vi "CAMcalibrator.vi"() -> ()   [LabVIEW 2011]
uses:
  <vilib>/userDefined/High Color/IMAQdx.ctl
  <vilib>/vision/driver/NI_Vision_Acquisition_Software.lvlib
panel:
  out "I (mA)":dbl
  out "Image":T1(plugin-control)
  in  "APTLaser":refnum<k7>(container) caption="Resume"
  in  "LaserON":bool
  in  "Set Current at:":sgl=70.0 caption="mA"
  in  "Parada Total":bool
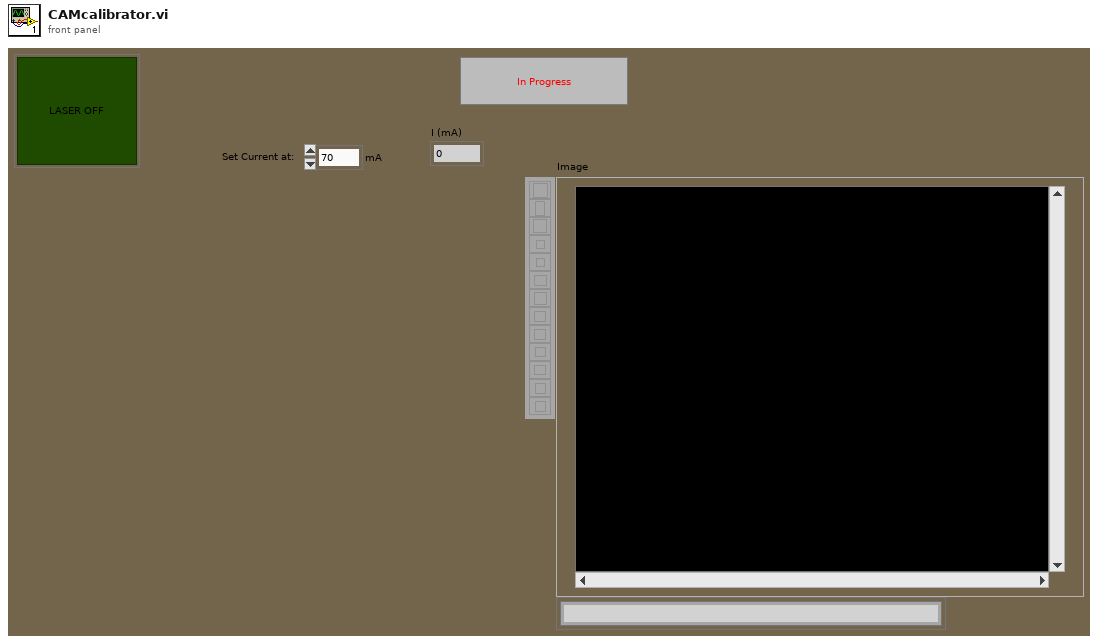
[diagram p1: front panel]
types:
  T1 = typedef "IMAQ Image.ctl" = refnum<image>
  T2 = typedef "IMAQdx.ctl" = refnum<k21>
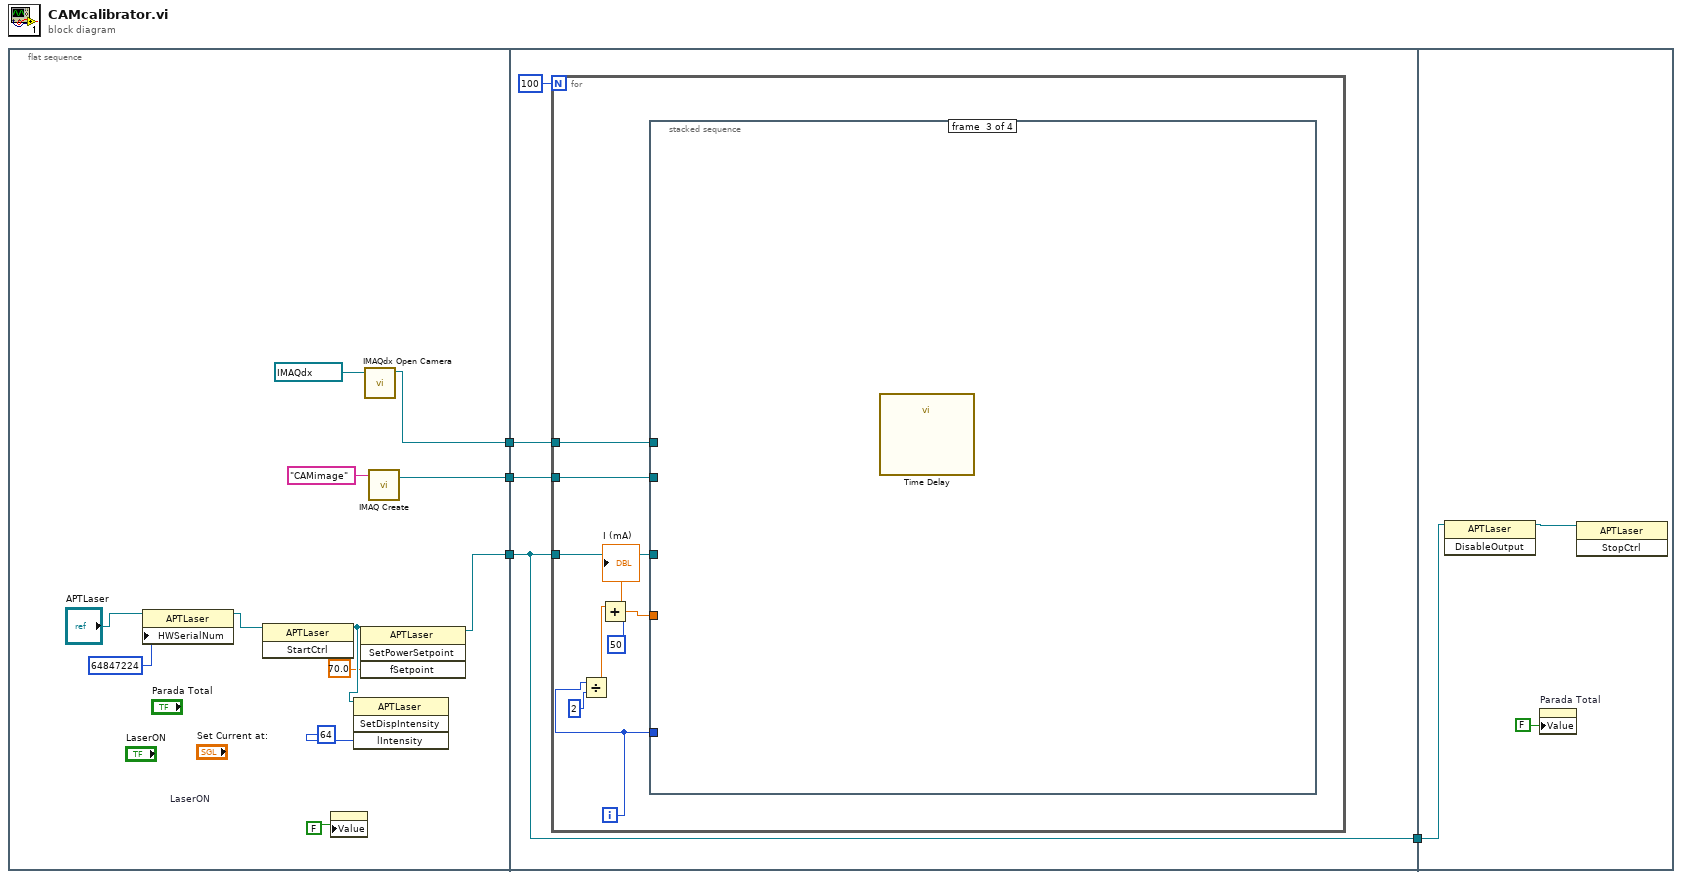
[diagram p0: block diagram]
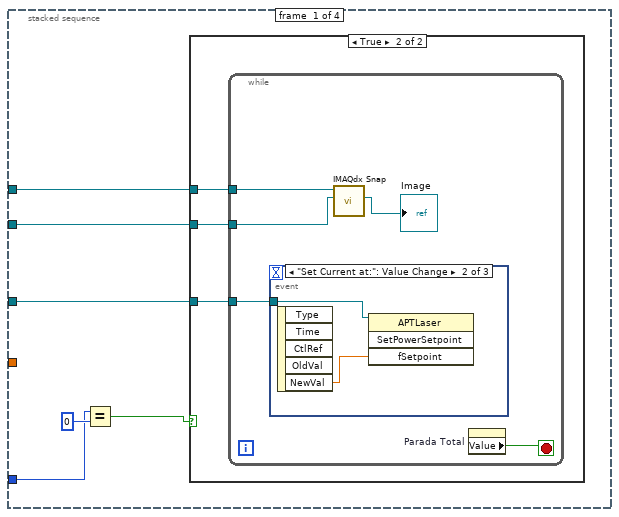
[diagram p2: hidden frame]
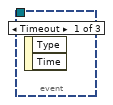
[diagram p4: hidden frame]
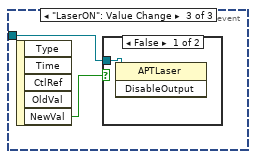
[diagram p5: hidden frame]
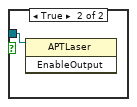
[diagram p6: hidden frame]
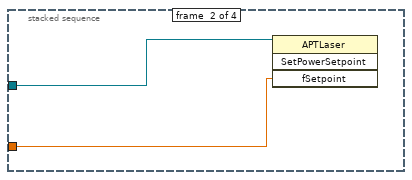
[diagram p7: hidden frame]
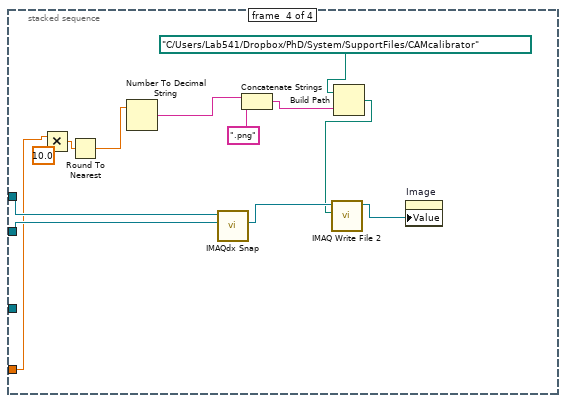
[diagram p8: hidden frame]
diagram:
  n1 = flat-sequence {
    tunnel: [w7] -> w4
    tunnel: [w6] -> w3
    tunnel: [w5] -> w2
    tunnel: w4 -> [w19]
    tunnel: w3 -> [w18]
    tunnel: w2 -> [w17]
    tunnel: [w17] -> w1
    tunnel: w1 -> [w65]
    frame #0 {
      n2 = property class="APTLaser"(reference="APTLaser", "HWSerialNum"=64847224) -> (reference out=w11:refnum<k7>)  [unwired: 1 in, 1 out]
      n3 = invoke class="APTLaser" method="StartCtrl"(reference=w11) -> (reference out=w16:refnum<k7>)  [unwired: 2 in, 2 out]
      n4 = property on="LaserON" class="Bool (strict)"("Value"=FALSE ("LaserON")) -> ()  [unwired: 2 in, 2 out]
      n5 = invoke class="APTLaser" method="SetDispIntensity"(reference=w16, "lIntensity"=64) -> ()  [unwired: 2 in, 4 out]
      n6 = invoke class="APTLaser" method="SetPowerSetpoint"(reference=w16, "fSetpoint"=sgl 70.0) -> (reference out=w5:refnum<k7>)  [unwired: 2 in, 3 out]
      n7 = call <vilib>:"IMAQdx Open Camera.vi"("Session In"=T2 "Paraxial") -> ("Session Out"=w7:T2)  [unwired: 9 in, 1 out]
      n8 = call "IMAQ Create"("Image Name"="CAMimage") -> ("New Image"=w6:T1)  [unwired: 4 in, 1 out]
    }
    frame #1 {
      n9 = for {
        N: 100 -> [_]
        tunnel: w19 -> [w28]
        tunnel: w18 -> [w27]
        tunnel: w17 -> [w26]
        i -> [w21]
        n10 = Divide(x=w21, y=2) -> (x/y=w25:dbl)
        n11 = Add(x=w25, y=50) -> (x+y=w22:dbl)
        "I (mA)" <- w22
        n12 = stacked-sequence {
          tunnel: w28 -> [w32 _ _ w63]
          tunnel: w27 -> [w31 _ _ w62]
          tunnel: w26 -> [w30 w50 _ _]
          tunnel: w22 -> [_ w49 _ w52]
          tunnel: w21 -> [w29 _ _ _]
          frame #0 {
            n13 = Equal?(x=w29, y=0) -> (x = y?=w33:bool)
            n14 = case shown="True" w33 {
              tunnel: w32 -> [_ w37]
              tunnel: w31 -> [_ w36]
              tunnel: w30 -> [_ w35]
              frame False {
              }
              frame True {
                n15 = while {
                  tunnel: w37 -> [w41]
                  tunnel: w36 -> [w40]
                  tunnel: w35 -> [w39]
                  stop <- w38 stop-if-true
                  n16 = event shown="[1] \"Set Current at:\": Value Change" {
                    selector: _ -> [_ _ _]
                    dyn-events: _ -> [_ _ _]
                    timeout: _ -> [_ _ _]
                    tunnel: w39 -> [_ w43 w45]
                    event Timeout {
                      n17 = event-data() -> ()  [unwired: 1 in, 2 out]
                    }
                    event "Set Current at:": Value Change {
                      n18 = event-data() -> ("NewVal"=w44:sgl)  [unwired: 1 in, 4 out]
                      n19 = invoke class="APTLaser" method="SetPowerSetpoint"(reference=w43, "fSetpoint"=w44) -> ()  [unwired: 2 in, 4 out]
                    }
                    event "LaserON": Value Change {
                      n20 = event-data() -> ("NewVal"=w46:bool)  [unwired: 1 in, 4 out]
                      n21 = case shown="False" w46 {
                        tunnel: w45 -> [w47 w48]
                        frame False {
                          n22 = invoke class="APTLaser" method="DisableOutput"(reference=w47) -> ()  [unwired: 2 in, 3 out]
                        }
                        frame True {
                          n23 = invoke class="APTLaser" method="EnableOutput"(reference=w48) -> ()  [unwired: 2 in, 3 out]
                        }
                      }
                    }
                  }
                  n24 = call <vilib>:"IMAQdx Snap.vi"("Image In"=w40, "Session In"=w41) -> ("Image Out"=→"Image":T1)  [unwired: 7 in, 2 out]
                  n25 = property on="Parada Total" class="Bool (strict)"() -> ("Value"=w38:bool)  [unwired: 2 in, 2 out]
                }
              }
            }
          }
          frame #1 {
            n26 = invoke class="APTLaser" method="SetPowerSetpoint"(reference=w50, "fSetpoint"=w49) -> ()  [unwired: 2 in, 4 out]
          }
          frame #2 {
            n27 = call "Time Delay"() -> ()  [unwired: 11 in, 1 out]
          }
          frame #3 {
            n28 = Multiply(x=w52, y=10.0) -> (x*y=w53:dbl)
            n29 = Round To Nearest(number=w53) -> (nearest integer value=w51:dbl)
            n30 = Number To Decimal String(number=w51) -> (decimal integer string=w57:string)  [unwired: 1 in]
            n31 = call <vilib>:"IMAQdx Snap.vi"("Image In"=w62, "Session In"=w63) -> ("Image Out"=w61:T1)  [unwired: 7 in, 2 out]
            n32 = Concatenate Strings(w57, ".png" ("string")) -> (w55:string)
            n33 = Build Path(base path=path "C:/Users/Lab541/Dropbox/PhD/System/SupportFiles/CAMcalibrator" ("File Path"), name or relative path=w55) -> (appended path=w58:path)
            n34 = call-poly "IMAQ Write File 2"("File Path"=w58, "Image"=w61) -> ("Image Out (duplicate)"=w60:T1)  [unwired: 8 in, 1 out]
            n35 = property on="Image" class="ImageControl"("Value"=w60) -> ()  [unwired: 2 in, 2 out]
          }
        }
      }
    }
    frame #2 {
      n36 = invoke class="APTLaser" method="DisableOutput"(reference=w65) -> (reference out=w66:refnum<k7>)  [unwired: 2 in, 2 out]
      n37 = property on="Parada Total" class="Bool (strict)"("Value"=FALSE ("Parada Total")) -> ()  [unwired: 2 in, 2 out]
      n38 = invoke class="APTLaser" method="StopCtrl"(reference=w66) -> ()  [unwired: 2 in, 3 out]
    }
  }
